vi "Open FPGA Session.vi"(7 "run when loaded (T)":bool=TRUE, 8 "error in":errorcluster, 10 "bitfile path":path, 11 "device address":string) -> (0 "error out":errorcluster, 2 "session out":u32, 3 "bitfile reference out":refnum<k20>)   [LabVIEW 2021, in "FPGA Register IO.lvlib"]
uses:
  FPGA Register IO.lvlib
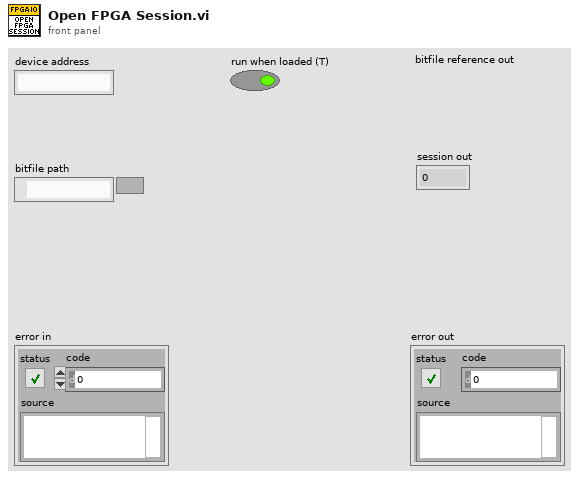
[diagram p1: front panel]
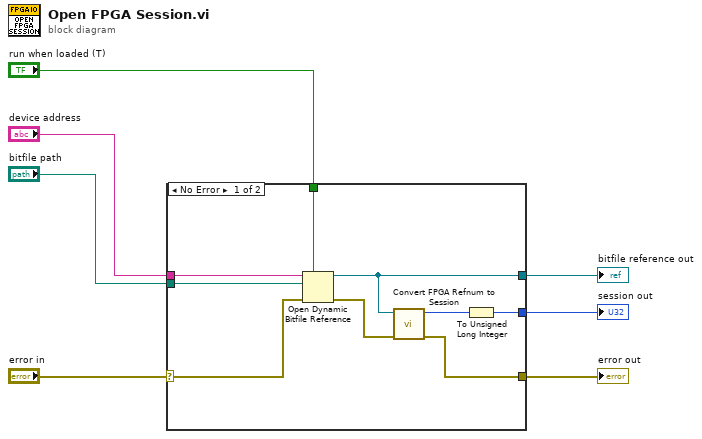
[diagram p0: block diagram]
diagram:
  n1 = case shown="No Error" "error in" {
    selector: "error in" -> [w12 w17]
    tunnel: "run when loaded (T)" -> [w16 _]
    tunnel: "device address" -> [w14 _]
    tunnel: "bitfile path" -> [w13 _]
    tunnel: [w11 w17] -> w3
    tunnel: [w10 _] -> w2
    tunnel: [w8 _] -> w1
    frame No Error {
      n2 = Open Dynamic Bitfile Reference(0:w14, 1:w13, 2:w16, 3:w12) -> (5:w10:refnum<k20>, 8:w15:errorcluster)  [unwired: 1 in]
      n3 = call "Convert FPGA Refnum to Session.vi"("error in (no error)"=w15, "fpga refnum in"=w10) -> ("error out"=w11:errorcluster, "session out"=w9:u64)  [unwired: 8 in]
      n4 = To Unsigned Long Integer(number=w9) -> (unsigned 32bit integer=w8:u32)
    }
    frame Error {
    }
  }
  "session out" <- w1
  "error out" <- w3
  "bitfile reference out" <- w2
